vi "Process.vi"(8 "error in":errorcluster, 11 "Plugin in":refnum<class "StreamWriter.lvclass">) -> (0 "error out":errorcluster, 3 "Plugin out":refnum<class "StreamWriter.lvclass">)   [LabVIEW 2024, in "StreamWriter.lvlib" / "StreamWriter.lvclass"]
uses:
  StreamWriter.lvclass
  StreamWriter.lvclass/StreamWriter.ctl
  <resource>/objmgr/ni.dex.rc
  <vilib>/FlexLogger/SDK/PluginSDK.lvlibp/PEFClasses/SDK/Plugin/Plugin.lvclass
  C:/Program Files/National Instruments/LabVIEW 2024/vi.lib/FlexLogger/SDK/PluginSDK.lvlibp/PEFClasses/SDK/Plugin/Plugin.lvclass
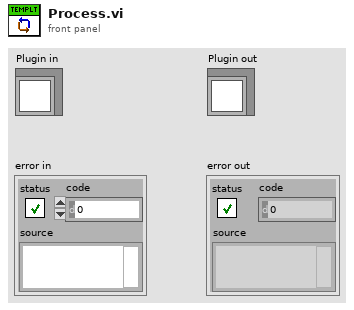
[diagram p1: front panel]
types:
  T1 = typedef "StreamWriter.lvlib/StreamWriter.lvclass/StreamWriter Parameters.ctl" = cluster{"Writer URL":string, "Timeout":i32, "Buffer Size":i32, "Writer Endpoint":refnum<k21>}
  T2 = cluster{"Data":waveform(dbl)[], "Stream Names":string[]}
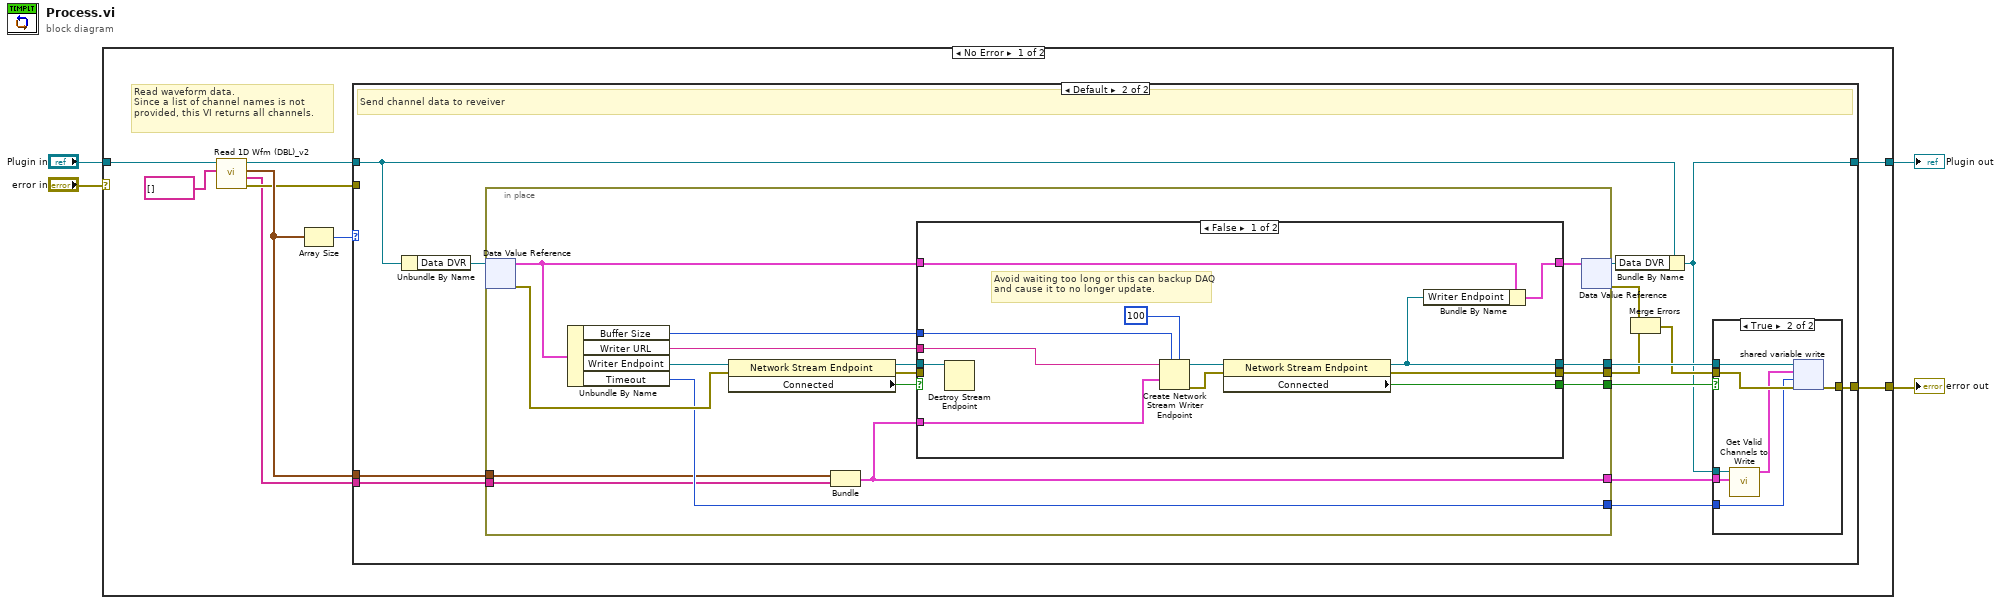
[diagram p0: block diagram]
diagram:
  n1 = case shown="No Error" "error in" {
    selector: "error in" -> [_ w69]
    tunnel: [w7 w70] -> w1
    tunnel: "Plugin in" -> [w5 w70]
    tunnel: [w6 w69] -> w2
    frame No Error {
      # "Read waveform data.\nSince a list of channel names is not provided, this VI returns all channels."
      n2 = call <vilib>:"Read 1D Wfm (DBL)_v2.vi"("Unique Identifers (empty = all)"=string[] [] ("Unique Channel Identifers (empty = all)"), "Plugin in"=w5) -> ("error out"=w10:errorcluster, "Stream Names"=w8:string[], "Data"=w13:waveform(dbl)[], "Plugin out"=w11:refnum<class "StreamWriter.lvclass">)  [unwired: 6 in]
      n3 = Array Size(array=w13) -> (size(s)=w12:i32)
      n4 = case shown="Default" w12 {
        tunnel: w13 -> [_ w19]
        tunnel: [w14 w29] -> w6
        tunnel: [w15 w16] -> w7
        tunnel: w11 -> [w15 w24]
        tunnel: w10 -> [w14 _]
        tunnel: w8 -> [_ w18]
        frame 0 {
          # "No channels sending data to the plugin"
        }
        frame Default {
          # "Send channel data to reveiver"
          n5 = Unbundle By Name(w24) -> ("Data DVR"=w26:refnum<data-value>)
          n6 = in-place {
            in-place-border: [w42] -> w22
            in-place-border: [w41] -> w28
            in-place-border: [w40] -> w27
            in-place-border: [w34] -> w20
            in-place-border: w19 -> [w33]
            in-place-border: w18 -> [w32]
            in-place-border: [w31] -> w17
            n7 = in-place-dvr #1(w26) -> (w37:T1, w35:errorcluster)
            n8 = Unbundle By Name(w37) -> ("Buffer Size"=w38:i32, "Writer URL"=w30:string, "Writer Endpoint"=w39:refnum<k21>, "Timeout"=w34:i32)
            n9 = property class="Network Stream Endpoint"(reference=w39, error in=w35) -> (reference out=w43:refnum<k21>, error out=w45:errorcluster, "Connected"=w44:bool)
            n10 = Bundle("Data"=w33, "Stream Names"=w32) -> (w31:T2)  [unwired: 1 in]
            n11 = case shown="False" w44 {
              selector: w44 -> [_ w59]
              tunnel: [w57 w58] -> w36
              tunnel: [w56 w60] -> w42
              tunnel: [w48 w61] -> w41
              tunnel: w43 -> [w55 w61]
              tunnel: [w54 w59] -> w40
              tunnel: w45 -> [_ w60]
              tunnel: w38 -> [w51 _]
              tunnel: w37 -> [w50 w58]
              tunnel: w31 -> [w49 _]
              tunnel: w30 -> [w47 _]
              frame False {
                # "Avoid waiting too long or this can backup DAQ and cause it to no longer update."
                n12 = Destroy Stream Endpoint(11:w55) -> ()  [unwired: 1 in, 1 out]
                n13 = Create Network Stream Writer Endpoint(5:100 ("timeout in ms (-1)"), 7:w51, 9:w49, 11:w47) -> (0:w52:errorcluster, 3:w53:refnum<k21>)  [unwired: 3 in]
                n14 = property class="Network Stream Endpoint"(reference=w53, error in=w52) -> (reference out=w48:refnum<k21>, error out=w56:errorcluster, "Connected"=w54:bool)
                n15 = Bundle By Name(cluster=w50, "Writer Endpoint"=w48) -> (w57:T1)
              }
              frame True {
              }
            }
            n16 = in-place-dvr #1(w36) -> (w23:refnum<data-value>, w25:errorcluster)
          }
          n17 = Bundle By Name(cluster=w24, "Data DVR"=w23) -> (w16:refnum<class "StreamWriter.lvclass">)
          n18 = Merge Errors(w25, w22) -> (w21:errorcluster)
          n19 = case shown="True" w27 {
            tunnel: w28 -> [_ w68]
            tunnel: w21 -> [_ w67]
            tunnel: [_ w66] -> w29
            tunnel: w17 -> [_ w64]
            tunnel: w20 -> [_ w65]
            tunnel: w16 -> [_ w62]
            frame False {
            }
            frame True {
              n20 = call "Get Valid Channels to Write.vi"("Data to Write In"=w64, "Plugin in"=w62) -> ("Data to Write Out"=w63:cluster{waveform(dbl)[], string[]})  [unwired: 8 in, 1 out]
              n21 = shared-variable-write(w68, w67, w63, w65) -> (w66:errorcluster)  [unwired: 2 out]
            }
          }
        }
      }
    }
    frame Error {
    }
  }
  "error out" <- w2
  "Plugin out" <- w1
